vi "Find-VIPath-from-CallChain.vi"(11 "Call Chain":string[](array[string])) -> (0 "error out":errorcluster, 2 "VI Path":path)   [LabVIEW 2020, in "Caraya.lvlib" / "Basic Test Manager.lvclass"]
uses:
  Basic Test Manager.lvclass
  Basic Test Manager.lvclass/Basic Test Manager.ctl
  <userlib>/_OpenG.lib/file/file.llb/openg_file.lvlib
  <userlib>/_OpenG.lib/file/file.llb/File Exists - Scalar__ogtk.vi
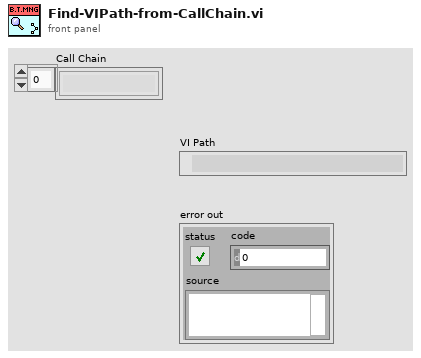
[diagram p1: front panel]
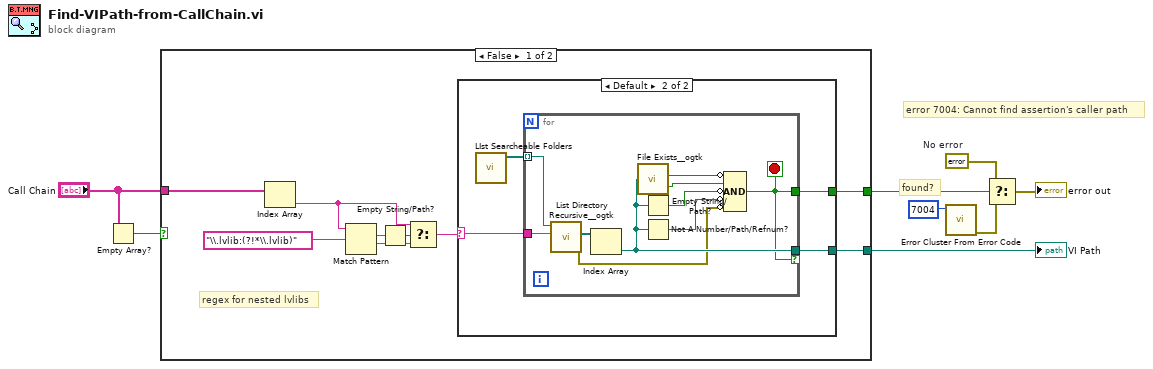
[diagram p0: block diagram]
diagram:
  w1 = errorcluster {"status"=FALSE, "code"=0, "source"=""}  # No error
  # "found?"
  # "error 7004: Cannot find assertion's caller path"
  n1 = Empty Array?(array="Call Chain") -> (empty?=w6:bool)
  n2 = case shown="False" w6 {
    tunnel: [w12 _] -> w8
    tunnel: "Call Chain" -> [w11 _]
    tunnel: [w9 _] -> w3
    frame False {
      # "regex for nested lvlibs"
      n3 = Index Array(array=w11) -> (element=w17:string)  [unwired: 1 in]
      n4 = Match Pattern(string=w17, regular expression="\\.lvlib:(?!*\\.lvlib)") -> (match substring=w14:string, after substring=w16:string)  [unwired: 1 in, 2 out]
      n5 = Empty String/Path?(string/path=w14) -> (empty?=w15:bool)
      n6 = Select(t=w17, s=w15, f=w16) -> (s? t:f=w10:string)
      n7 = case shown="Default" w10 {
        selector: w10 -> [_ w20]
        tunnel: [_ w21] -> w12
        tunnel: [_ w19] -> w9
        frame "" {
        }
        frame Default {
          n8 = call "LIst Searcheable Folders.vi"() -> ("Searcheable Folders"=w18:path[])  [unwired: 11 in]
          n9 = for {
            tunnel: [w31] -> w21 if=w22
            tunnel: w20 -> [w30]
            tunnel: [w22] -> w19
            tunnel: w18 -> [w29] mode=indexing
            stop <- w22 stop-if-true
            n10 = call <userlib>:"List Directory Recursive__ogtk.vi"("pattern"=w30, "Path"=w29) -> ("error out"=w23:errorcluster, "file paths"=w28:path[])  [unwired: 6 in, 2 out]
            n11 = Index Array(array=w28) -> (element=w31:path)  [unwired: 1 in]
            n12 = call-poly <userlib>:"File Exists__ogtk.vi"("file path"=w31) -> ("is directory"=w27:bool, "exists"=w26:bool)  [unwired: 6 in]
            n13 = Empty String/Path?(string/path=w31) -> (empty?=w25:bool)
            n14 = Not A Number/Path/Refnum?(number/path/refnum=w31) -> (NaN/Path/Refnum?=w24:bool)
            n15 = Compound Arithmetic op=AND(invert w27, w26, invert w25, invert w24, invert w23) -> (w22:bool)
          }
        }
      }
    }
    frame True {
    }
  }
  "VI Path" <- w8
  n16 = call <vilib>:"Error Cluster From Error Code.vi"("error code (0)"=7004) -> ("error out"=w2:errorcluster)  [unwired: 8 in]
  n17 = Select(t=w1, s=w3, f=w2) -> (s? t:f=→"error out":errorcluster)
